vi "Read RF Marker Values.vi"(0 "VISA resource name":refnum<visa-resource-name>, 11 "error in (no error)":errorcluster) -> (4 "VISA resource name out":refnum<visa-resource-name>, 6 "Reference Peak Array":dbl[](array[numeric]), 8 "Manual Marker Array":dbl[][](array[numeric]), 10 "Auto Peak Array":dbl[][](array[numeric]), 15 "error out":errorcluster)   [LabVIEW 2016, in "Tektronix DPO MSO 2000 4000 Series.lvlib"]
doc: "Reads the values of the various markers that have been placed on the frequency domain. These markers return information such as the frequency and amplitude for markers as well as read peak information.\n\n<B>Note:</B>\nOnly valid on <B>MDO</B> series oscilliscopes."
uses:
  Tektronix DPO MSO 2000 4000 Series.lvlib
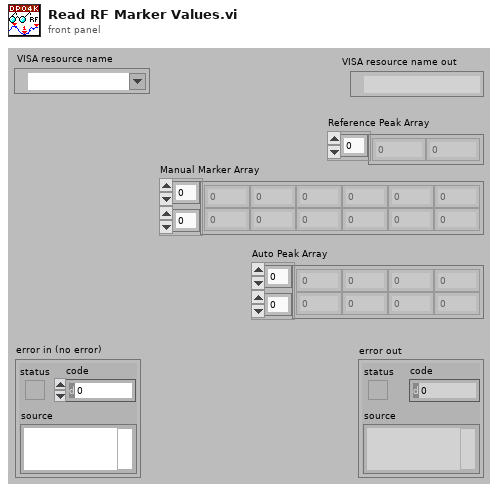
[diagram p1: front panel]
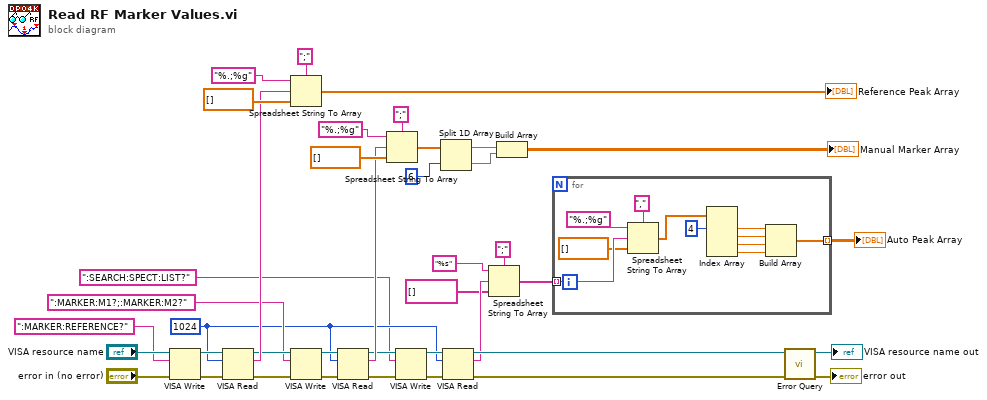
[diagram p0: block diagram]
diagram:
  w10 = u32 1024 ("byte count")
  n1 = VISA Write(VISA resource name="VISA resource name", write buffer=":MARKER:REFERENCE?", error in (no error)="error in (no error)") -> (VISA resource name out=w35:refnum<visa-resource-name>, error out=w36:errorcluster)  [unwired: 1 out]
  n2 = VISA Read(VISA resource name=w35, byte count=w10, error in (no error)=w36) -> (VISA resource name out=w27:refnum<visa-resource-name>, read buffer=w28:string, error out=w29:errorcluster)  [unwired: 1 out]
  n3 = Spreadsheet String To Array(delimiter (Tab)=";", format string="%.;%g", spreadsheet string=w28, array type (2D Dbl)=dbl[] []) -> (array=→"Reference Peak Array":dbl[])
  n4 = VISA Write(VISA resource name=w27, write buffer=":MARKER:M1?;:MARKER:M2?", error in (no error)=w29) -> (VISA resource name out=w24:refnum<visa-resource-name>, error out=w25:errorcluster)  [unwired: 1 out]
  n5 = VISA Read(VISA resource name=w24, byte count=w10, error in (no error)=w25) -> (VISA resource name out=w11:refnum<visa-resource-name>, read buffer=w12:string, error out=w13:errorcluster)  [unwired: 1 out]
  n6 = Spreadsheet String To Array(delimiter (Tab)=";", format string="%.;%g", spreadsheet string=w12, array type (2D Dbl)=dbl[] []) -> (array=w20:dbl[])
  n7 = VISA Write(VISA resource name=w11, write buffer=":SEARCH:SPECT:LIST?", error in (no error)=w13) -> (VISA resource name out=w15:refnum<visa-resource-name>, error out=w14:errorcluster)  [unwired: 1 out]
  n8 = Split 1D Array(array=w20, index=6) -> (first subarray=w18:dbl[], second subarray=w17:dbl[])
  n9 = VISA Read(VISA resource name=w15, byte count=w10, error in (no error)=w14) -> (VISA resource name out=w9:refnum<visa-resource-name>, read buffer=w7:string, error out=w8:errorcluster)  [unwired: 1 out]
  n10 = Spreadsheet String To Array(delimiter (Tab)=";", format string="%s", spreadsheet string=w7, array type (2D Dbl)=string[] []) -> (array=w3:string[])
  n11 = Build Array(w18, w17) -> (→"Manual Marker Array":dbl[][])
  n12 = for {
    tunnel: [w46] -> w1 mode=indexing
    tunnel: w3 -> [w44] mode=indexing
    n13 = Spreadsheet String To Array(delimiter (Tab)=",", format string="%.;%g", spreadsheet string=w44, array type (2D Dbl)=dbl[] []) -> (array=w45:dbl[])
    n14 = Index Array(array=w45, index #1=4 ("index")) -> (element #1=w47:dbl, element #2=w48:dbl, element #3=w49:dbl, element #4=w50:dbl)  [unwired: 3 in]
    n15 = Build Array(w47, w48, w49, w50) -> (w46:dbl[])
  }
  "Auto Peak Array" <- w1
  n16 = call "Error Query.vi"("error in (no error)"=w8, "VISA resource name"=w9) -> ("error out"=→"error out":errorcluster, "VISA resource name out"=→"VISA resource name out":refnum<visa-resource-name>)  [unwired: 6 in, 2 out]
